vi "EnableAllNotifications.vi"(6 "Connection Status":T1={"MAC Address"="", "cnx handle"=0, "cnx flags"=0, "Address Type"=125, "Connection Interval (ms)"=125, "Timeout(ms)"=125, "Latency"=0, "bonding handle"=0} {"Address Type" items=["Public", "Random"]}, 7 "Handle table":string[][](array[string]), 8 "error in":errorcluster, 10 "1 or 0":u16=1, 11 "COM Bluegiga in":refnum<visa-resource-name>) -> (0 "error out":errorcluster, 3 "COM Bluegiga out":refnum<visa-resource-name>)   [LabVIEW 2015]
uses:
  <vilib>/BLE/type_def/connection_status_bundle.ctl
  <vilib>/BLE/type_def/address_type.ctl
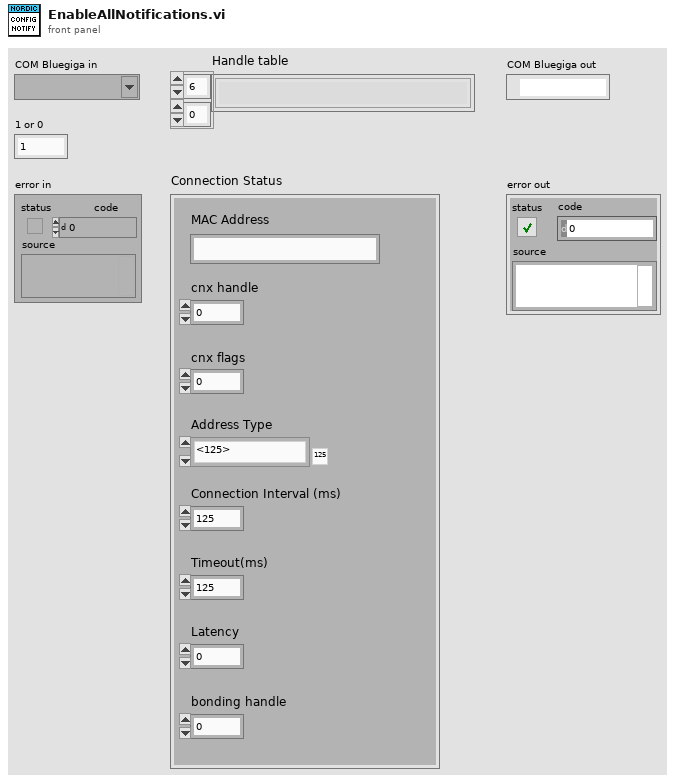
[diagram p1: front panel]
types:
  T1 = typedef "connection_status_bundle.ctl" = cluster{"MAC Address":string, "cnx handle":u8, "cnx flags":u8, "Address Type":T2, "Connection Interval (ms)":u16, "Timeout(ms)":u16, "Latency":u16, "bonding handle":u8}
  T2 = typedef "address_type.ctl" = u8
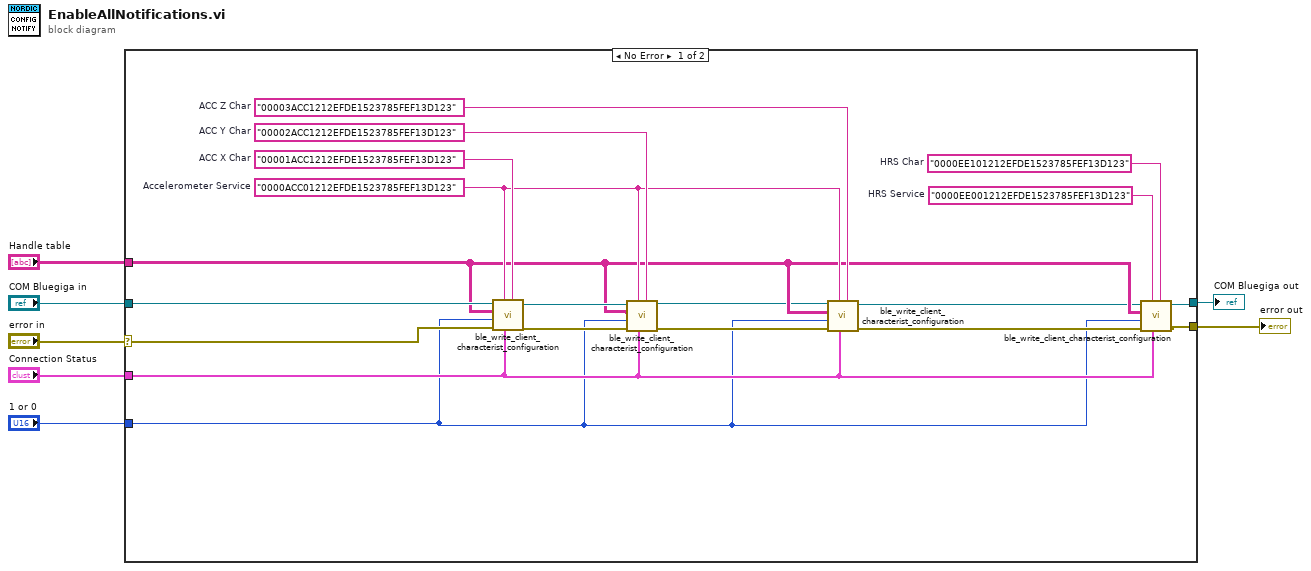
[diagram p0: block diagram]
diagram:
  n1 = case shown="No Error" "error in" {
    selector: "error in" -> [w24 w27]
    tunnel: "Connection Status" -> [w15 _]
    tunnel: "Handle table" -> [w18 _]
    tunnel: "COM Bluegiga in" -> [w25 _]
    tunnel: [w11 w27] -> w2
    tunnel: [w12 _] -> w3
    tunnel: "1 or 0" -> [w8 _]
    frame No Error {
      w9 = "0000EE101212EFDE1523785FEF13D123"  # HRS Char
      w10 = "0000EE001212EFDE1523785FEF13D123"  # HRS Service
      w19 = "00003ACC1212EFDE1523785FEF13D123"  # ACC Z Char
      w23 = "00002ACC1212EFDE1523785FEF13D123"  # ACC Y Char
      w26 = "00001ACC1212EFDE1523785FEF13D123"  # ACC X Char
      w20 = "0000ACC01212EFDE1523785FEF13D123"  # Accelerometer Service
      n2 = call <vilib>:"ble_write_client_characterist_configuration.vi"("Characteristic UUID"=w26, "Connection Status"=w15, "Service UUID"=w20, "error in (no error)"=w24, "Value(16bit)"=w8, "Handle table"=w18, "COM Bluegiga in"=w25) -> ("error out"=w21:errorcluster, "COM Bluegiga out"=w22:refnum<visa-resource-name>)  [unwired: 3 in]
      n3 = call <vilib>:"ble_write_client_characterist_configuration.vi"("Characteristic UUID"=w23, "Connection Status"=w15, "Service UUID"=w20, "error in (no error)"=w21, "Value(16bit)"=w8, "Handle table"=w18, "COM Bluegiga in"=w22) -> ("error out"=w16:errorcluster, "COM Bluegiga out"=w17:refnum<visa-resource-name>)  [unwired: 3 in]
      n4 = call <vilib>:"ble_write_client_characterist_configuration.vi"("Characteristic UUID"=w19, "Connection Status"=w15, "Service UUID"=w20, "error in (no error)"=w16, "Value(16bit)"=w8, "Handle table"=w18, "COM Bluegiga in"=w17) -> ("error out"=w13:errorcluster, "COM Bluegiga out"=w14:refnum<visa-resource-name>)  [unwired: 3 in]
      n5 = call <vilib>:"ble_write_client_characterist_configuration.vi"("Characteristic UUID"=w9, "Connection Status"=w15, "Service UUID"=w10, "error in (no error)"=w13, "Value(16bit)"=w8, "Handle table"=w18, "COM Bluegiga in"=w14) -> ("error out"=w11:errorcluster, "COM Bluegiga out"=w12:refnum<visa-resource-name>)  [unwired: 3 in]
    }
    frame Error {
    }
  }
  "COM Bluegiga out" <- w3
  "error out" <- w2
